vi "PCACompute.vi"(8 "error in":errorcluster, 10 "maxComponents":i32, 11 "Data":dbl[][](array[numeric])) -> (0 "error out":errorcluster, 1 "EigenValues":dbl[](array[numeric]), 2 "EigenVectors":dbl[][](array[numeric]), 3 "Mean":dbl[][](array[numeric]))   [LabVIEW 2020, in "OpenLvVision_OpenCv.lvlib"]
doc: "Performs PCA of the supplied dataset."
uses:
  _LvHelpers/MatHandling/RegisterMat/RegisterMat_Array2D-DBL.vi
  _LvHelpers/MatHandling/UnregisterMat/UnregisterMat_2DArray-DBL.vi
  OpenLvVision_OpenCv.lvlib
  Dlls/OlvOpenCvWrapper.dll
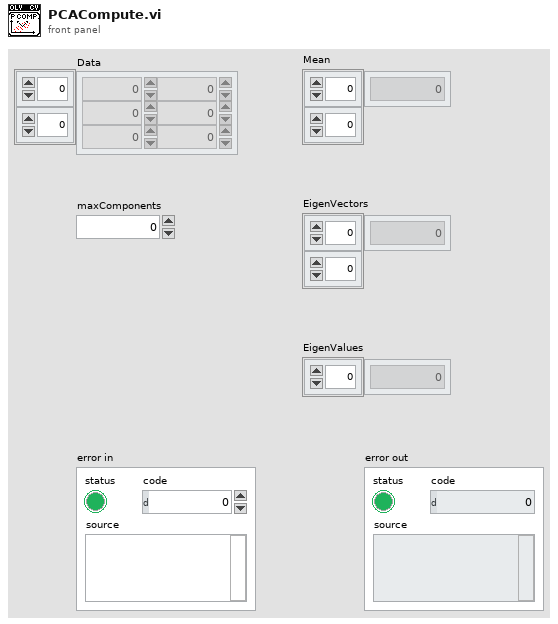
[diagram p1: front panel]
types:
  T1 = typedef "OpenLvVision_OpenCv.lvlib/MatInfo.ctl" = cluster{"Datatype":T2, "Height":i32, "Width":i32, "Channels":i32, "LineWidth":i32, "Null":u8}
  T2 = typedef "OpenLvVision_OpenCv.lvlib/LvDatatype.ctl" = enum32{"Undefined", "U8", "I8", "U16", "I16", "U32_Color", "I32", "U64_Color", "I64", "SGL", "DBL", "Complex SGL", "Complex DBL", "Array 1D U8", "Array 1D I8", "Array 1D U16", "Array 1D I16", "Array 1D U32_Color", "Array 1D I32", "Array 1D U64_Color", "Array 1D I64", "Array 1D SGL", "Array 1D DBL", "Array 1D Complex SGL", "Array 1D Complex DBL", "Array 2D U8", "Array 2D I8", "Array 2D U16", "Array 2D I16", "Array 2D U32", "Array 2D U32_Color", "Array 2D I32", "Array 2D U64", "Array 2D U64_Color", "Array 2D I64", "Array 2D SGL", "Array 2D DBL", "Array 2D Complex SGL", "Array 2D Complex DBL", "Image Mono U8", "Image Mono U16", "Image Mono I16", "Image Mono SGL", "Image Color U32", "Image Color U64", "ImageComplex Sgl", "Array1d_2dPointI32", "Array1d_2dPointSGL", "Array1d_2dPointDBL", "Array1d_3dPointI32", "Array1d_3dPointSGL", "Array1d_3dPointDBL", "Array1d_4dPointI32", "Array1d_4dPointSGL", "Array1d_4dPointDBL"}
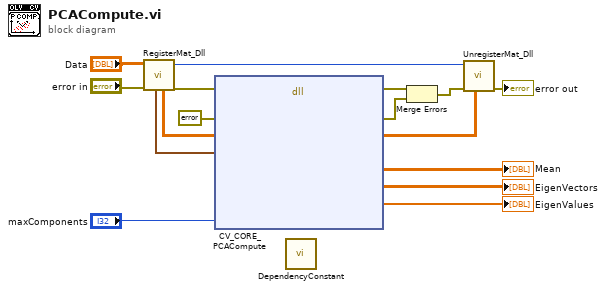
[diagram p0: block diagram]
diagram:
  n1 = call-poly "RegisterMat_Dll.vi"("error in"="error in", "Array in"="Data") -> ("error out"=w15:errorcluster, "Image"=w13:u8, "AdressOrData"=w12:dbl[][], "Mat"=w11:T1)  [unwired: 6 in]
  n2 = dll-call lib="C:/Users/lukas/Downloads/OpenLvVision_OpenCv/SourceCode/LabView/OpenLvVision_OpenCv/Dlls/OlvOpenCvWrapper.dll" fn="CV_CORE_PCACompute"(error in=w15, "Error"=errorcluster {"status"=FALSE, "code"=0, "source"=""} ("error constant"), "AdressData"=w12, "MatInfoData"=w11, "maxComponents"="maxComponents") -> (error out=w7:errorcluster, "Error"=w6:errorcluster, "AdressData"=w10:dbl[][], "mean"=→"Mean":dbl[][], "eigenvectors"=→"EigenVectors":dbl[][], "eigenvalues"=→"EigenValues":dbl[])  [unwired: 8 in, 1 out]
  n3 = call "DependencyConstant.vi"() -> ()  [unwired: 12 in]
  n4 = Merge Errors(w7, w6) -> (w5:errorcluster)
  n5 = call-poly "UnregisterMat_Dll.vi"("AdressOrData"=w10, "error in"=w5, "Image"=w13) -> ("error out"=→"error out":errorcluster)  [unwired: 7 in, 1 out]
